vi "NI-DCPower Advanced Sequence Retrigger.vi"() -> ()   [LabVIEW 2023]
doc: "Demonstrates how to use the Advanced Sequence functions to change the output function in a sequence. This example initializes a session, configures the Source Delay, creates an Advanced Sequence, creates a step to set the configured Voltage Level in DC Voltage mode, creates a step to set the configured Current Level in DC Current mode, initiates generation, waits for a specified delay, and measures the voltage and current output. This example uses Advanced Sequence source mode."
uses:
  AdvancedSequenceSettings.ctl
  AdancedLCRSeqAppCluster.ctl
  MessageDef.ctl
  <instrlib>/niDCPower/nidcpower.llb/niDCPower Source Mode.ctl
  <instrlib>/niDCPower/nidcpower.llb/niDCPower Wait For Event - Event.ctl
  <instrlib>/niDCPower/nidcpower.llb/niDCPower Send Software Edge Trigger - Signal.ctl
  <instrlib>/niDCPower/nidcpower.llb/niDCPower Get Channel Name From String.vi
  <instrlib>/niDCPower/nidcpower.llb/niDCPower Configure Software Edge Start Trigger With Channels.vi
panel:
  in  "Combo Box":string(combo)="Mixed"
  in  "Trigger":bool
  in  "Stop":bool
  in  "Hardware timed Instrument Settings Inital Setup":T1[](array[typedef])=[{"Sequence Name"="LCRSweep_Low", "SequenceSettings"=[{"Instrument Mode"=1062, "LCR:AC Stimulus:Voltage Amplitude"=0.1, "LCR:AC Stimulus:Frequency"=1000.0, "Source:DC Voltage:Voltage Level"=0.0, "Source:DC Voltage:Current Limit"=0.001}, {"Instrument Mode"=1062, "LCR:AC Stimulus:Voltage Amplitude"=0.15, "LCR:AC Stimulus:Frequency"=2000.0, "Source:DC Voltage:Voltage Level"=0.0, "Source:DC Voltage:Current Limit"=0.001}, {"Instrument Mode"=1062, "LCR:AC Stimulus:Voltage Amplitude"=0.1, "LCR:AC Stimulus:Frequency"=2000.0, "Source:DC Voltage:Voltage Level"=0.0, "Source:DC Voltage:Current Limit"=1e-05}, {"Instrument Mode"=1062, "LCR:AC Stimulus:Voltage Amplitude"=0.1, "LCR:AC Stimulus:Frequency"=2000.0, "Source:DC Voltage:Voltage Level"=4.0, "Source:DC Voltage:Current Limit"=1e-05}, {"Instrument Mode"=1062, "LCR:AC Stimulus:Voltage Amplitude"=0.2, "LCR:AC Stimulus:Frequency"=2000.0, "Source:DC Voltage:Voltage Level"=3.0, "Source:DC Voltage:Current Limit"=1e-05}, {"Instrument Mode"=1062, "LCR:AC Stimulus:Voltage Amplitude"=1.0, "LCR:AC Stimulus:Frequency"=5000.0, "Source:DC Voltage:Voltage Level"=1.0, "Source:DC Voltage:Current Limit"=1e-05}]}, {"Sequence Name"="LCRSweep_High", "SequenceSettings"=[{"Instrument Mode"=1062, "LCR:AC Stimulus:Voltage Amplitude"=5.0, "LCR:AC Stimulus:Frequency"=1000.0, "Source:DC Voltage:Voltage Level"=0.0, "Source:DC Voltage:Current Limit"=0.001}, {"Instrument Mode"=1062, "LCR:AC Stimulus:Voltage Amplitude"=4.0, "LCR:AC Stimulus:Frequency"=2000.0, "Source:DC Voltage:Voltage Level"=0.0, "Source:DC Voltage:Current Limit"=0.001}, {"Instrument Mode"=1062, "LCR:AC Stimulus:Voltage Amplitude"=1.0, "LCR:AC Stimulus:Frequency"=2000.0, "Source:DC Voltage:Voltage Level"=0.0, "Source:DC Voltage:Current Limit"=1e-05}, {"Instrument Mode"=1062, "LCR:AC Stimulus:Voltage Amplitude"=1.5, "LCR:AC Stimulus:Frequency"=2000.0, "Source:DC Voltage:Voltage Level"=4.0, "Source:DC Voltage:Current Limit"=1e-05}, {"Instrument Mode"=1062, "LCR:AC Stimulus:Voltage Amplitude"=4.0, "LCR:AC Stimulus:Frequency"=2000.0, "Source:DC Voltage:Voltage Level"=3.0, "Source:DC Voltage:Current Limit"=1e-05}, {"Instrument Mode"=1062, "LCR:AC Stimulus:Voltage Amplitude"=3.0, "LCR:AC Stimulus:Frequency"=5000.0, "Source:DC Voltage:Voltage Level"=1.0, "Source:DC Voltage:Current Limit"=1e-05}]}, {"Sequence Name"="MixedModes", "SequenceSettings"=[{"Instrument Mode"=1062, "LCR:AC Stimulus:Voltage Amplitude"=1.0, "LCR:AC Stimulus:Frequency"=1000.0, "Source:DC Voltage:Voltage Level"=0.0, "Source:DC Voltage:Current Limit"=0.001}, {"Instrument Mode"=1061, "LCR:AC Stimulus:Voltage Amplitude"=0.15, "LCR:AC Stimulus:Frequency"=2000.0, "Source:DC Voltage:Voltage Level"=3.0, "Source:DC Voltage:Current Limit"=0.001}, {"Instrument Mode"=1062, "LCR:AC Stimulus:Voltage Amplitude"=1.0, "LCR:AC Stimulus:Frequency"=2000.0, "Source:DC Voltage:Voltage Level"=0.0, "Source:DC Voltage:Current Limit"=1e-05}, {"Instrument Mode"=1061, "LCR:AC Stimulus:Voltage Amplitude"=0.1, "LCR:AC Stimulus:Frequency"=2000.0, "Source:DC Voltage:Voltage Level"=2.0, "Source:DC Voltage:Current Limit"=1e-05}, {"Instrument Mode"=1062, "LCR:AC Stimulus:Voltage Amplitude"=0.2, "LCR:AC Stimulus:Frequency"=2000.0, "Source:DC Voltage:Voltage Level"=3.0, "Source:DC Voltage:Current Limit"=1e-05}, {"Instrument Mode"=1062, "LCR:AC Stimulus:Voltage Amplitude"=1.0, "LCR:AC Stimulus:Frequency"=5000.0, "Source:DC Voltage:Voltage Level"=1.0, "Source:DC Voltage:Current Limit"=1e-05}]}, {"Sequence Name"="SMU_Low", "SequenceSettings"=[{"Instrument Mode"=1062, "LCR:AC Stimulus:Voltage Amplitude"=0.1, "LCR:AC Stimulus:Frequency"=1000.0, "Source:DC Voltage:Voltage Level"=0.0, "Source:DC Voltage:Current Limit"=0.001}, {"Instrument Mode"=1062, "LCR:AC Stimulus:Voltage Amplitude"=0.15, "LCR:AC Stimulus:Frequency"=2000.0, "Source:DC Voltage:Voltage Level"=1.0, "Source:DC Voltage:Current Limit"=0.001}, {"Instrument Mode"=1062, "LCR:AC Stimulus:Voltage Amplitude"=0.1, "LCR:AC Stimulus:Frequency"=2000.0, "Source:DC Voltage:Voltage Level"=0.0, "Source:DC Voltage:Current Limit"=1e-05}, {"Instrument Mode"=1062, "LCR:AC Stimulus:Voltage Amplitude"=0.1, "LCR:AC Stimulus:Frequency"=2000.0, "Source:DC Voltage:Voltage Level"=2.0, "Source:DC Voltage:Current Limit"=1e-05}, {"Instrument Mode"=1061, "LCR:AC Stimulus:Voltage Amplitude"=0.2, "LCR:AC Stimulus:Frequency"=2000.0, "Source:DC Voltage:Voltage Level"=1.0, "Source:DC Voltage:Current Limit"=1e-05}, {"Instrument Mode"=1062, "LCR:AC Stimulus:Voltage Amplitude"=1.0, "LCR:AC Stimulus:Frequency"=5000.0, "Source:DC Voltage:Voltage Level"=1.0, "Source:DC Voltage:Current Limit"=1e-05}]}, {"Sequence Name"="SMU_High", "SequenceSettings"=[{"Instrument Mode"=1062, "LCR:AC Stimulus:Voltage Amplitude"=0.1, "LCR:AC Stimulus:Frequency"=1000.0, "Source:DC Voltage:Voltage Level"=3.0, "Source:DC Voltage:Current Limit"=0.001}, {"Instrument Mode"=1061, "LCR:AC Stimulus:Voltage Amplitude"=0.15, "LCR:AC Stimulus:Frequency"=2000.0, "Source:DC Voltage:Voltage Level"=2.0, "Source:DC Voltage:Current Limit"=0.001}, {"Instrument Mode"=1062, "LCR:AC Stimulus:Voltage Amplitude"=0.1, "LCR:AC Stimulus:Frequency"=2000.0, "Source:DC Voltage:Voltage Level"=6.0, "Source:DC Voltage:Current Limit"=1e-05}, {"Instrument Mode"=1062, "LCR:AC Stimulus:Voltage Amplitude"=0.1, "LCR:AC Stimulus:Frequency"=2000.0, "Source:DC Voltage:Voltage Level"=10.0, "Source:DC Voltage:Current Limit"=1e-05}, {"Instrument Mode"=1062, "LCR:AC Stimulus:Voltage Amplitude"=0.2, "LCR:AC Stimulus:Frequency"=2000.0, "Source:DC Voltage:Voltage Level"=7.0, "Source:DC Voltage:Current Limit"=1e-05}, {"Instrument Mode"=1062, "LCR:AC Stimulus:Voltage Amplitude"=1.0, "LCR:AC Stimulus:Frequency"=5000.0, "Source:DC Voltage:Voltage Level"=8.0, "Source:DC Voltage:Current Limit"=1e-05}]}, {"Sequence Name"="MixedMode_2", "SequenceSettings"=[{"Instrument Mode"=1062, "LCR:AC Stimulus:Voltage Amplitude"=0.1, "LCR:AC Stimulus:Frequency"=1000.0, "Source:DC Voltage:Voltage Level"=0.0, "Source:DC Voltage:Current Limit"=0.001}, {"Instrument Mode"=1062, "LCR:AC Stimulus:Voltage Amplitude"=0.15, "LCR:AC Stimulus:Frequency"=2000.0, "Source:DC Voltage:Voltage Level"=0.0, "Source:DC Voltage:Current Limit"=0.001}, {"Instrument Mode"=1061, "LCR:AC Stimulus:Voltage Amplitude"=0.1, "LCR:AC Stimulus:Frequency"=2000.0, "Source:DC Voltage:Voltage Level"=0.0, "Source:DC Voltage:Current Limit"=1e-05}, {"Instrument Mode"=1062, "LCR:AC Stimulus:Voltage Amplitude"=0.1, "LCR:AC Stimulus:Frequency"=2000.0, "Source:DC Voltage:Voltage Level"=4.0, "Source:DC Voltage:Current Limit"=1e-05}, {"Instrument Mode"=1061, "LCR:AC Stimulus:Voltage Amplitude"=0.2, "LCR:AC Stimulus:Frequency"=2000.0, "Source:DC Voltage:Voltage Level"=3.0, "Source:DC Voltage:Current Limit"=1e-05}, {"Instrument Mode"=1062, "LCR:AC Stimulus:Voltage Amplitude"=1.0, "LCR:AC Stimulus:Frequency"=5000.0, "Source:DC Voltage:Voltage Level"=1.0, "Source:DC Voltage:Current Limit"=1e-05}]}] {"SequenceSettings"."Instrument Mode" items=["SMU PS"=1061, "LCR"=1062, "E-Load"=1154]}
  out "error out":errorcluster
  out "Data":T2(graph)
  in  "Resource Name":refnum<k15>="SMU_4139_C02_S02"
  # "This Demo shows the reuse of Advanced Hardware timed sequences. In the Array on the left side the Sequences are defined and loaded\nWhile the Application is running you can then trigger these Sequences by Selecting the Sequence in the Combobox and press the Trigger Button."
  # "Init Application"
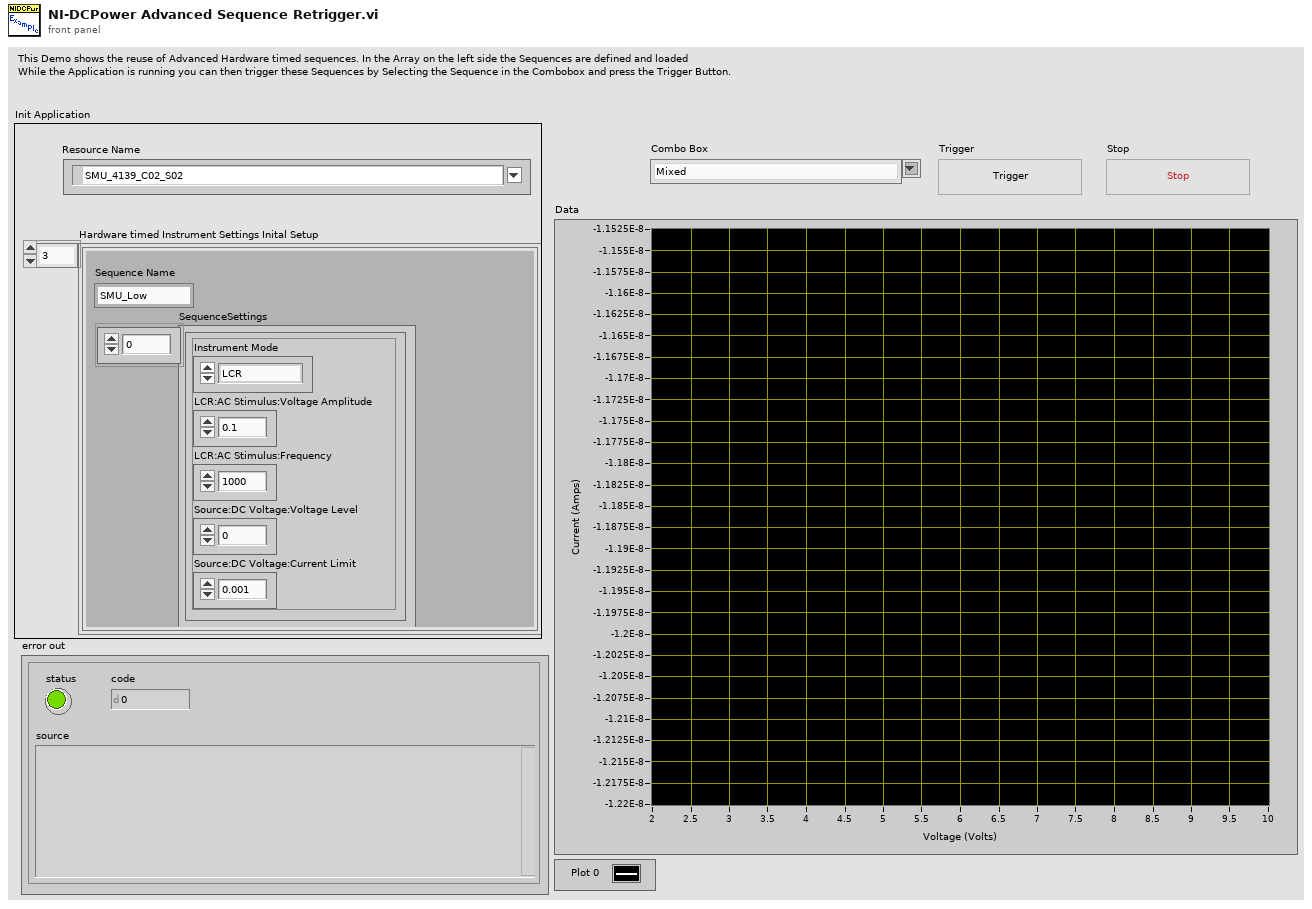
[diagram p1: front panel]
types:
  T1 = typedef "AdvancedSequenceSettings.ctl" = cluster{"Sequence Name":string, "SequenceSettings":cluster{"Instrument Mode":i32, "LCR:AC Stimulus:Voltage Amplitude":dbl, "LCR:AC Stimulus:Frequency":dbl, "Source:DC Voltage:Voltage Level":dbl, "Source:DC Voltage:Current Limit":dbl}[]}
  T2 = cluster{"voltage measurements":dbl[], "current measurements":dbl[]}
  T3 = typedef "AdancedLCRSeqAppCluster.ctl" = cluster{"queue out":refnum<queue>, "sequence name":string[], "Channelname":string, "instrument handle out":refnum<k15>}
  T4 = typedef "MessageDef.ctl" = cluster{"Message":string, "Data":variant}
  T5 = typedef "niDCPower Source Mode.ctl" = i32
  T6 = typedef "niDCPower Send Software Edge Trigger - Signal.ctl" = i32
  T7 = typedef "niDCPower Wait For Event - Event.ctl" = i32
  T8 = cluster{"Instrument Mode":i32, "LCR:AC Stimulus:Voltage Amplitude":dbl, "LCR:AC Stimulus:Frequency":dbl, "Source:DC Voltage:Voltage Level":dbl, "Source:DC Voltage:Current Limit":dbl}[]
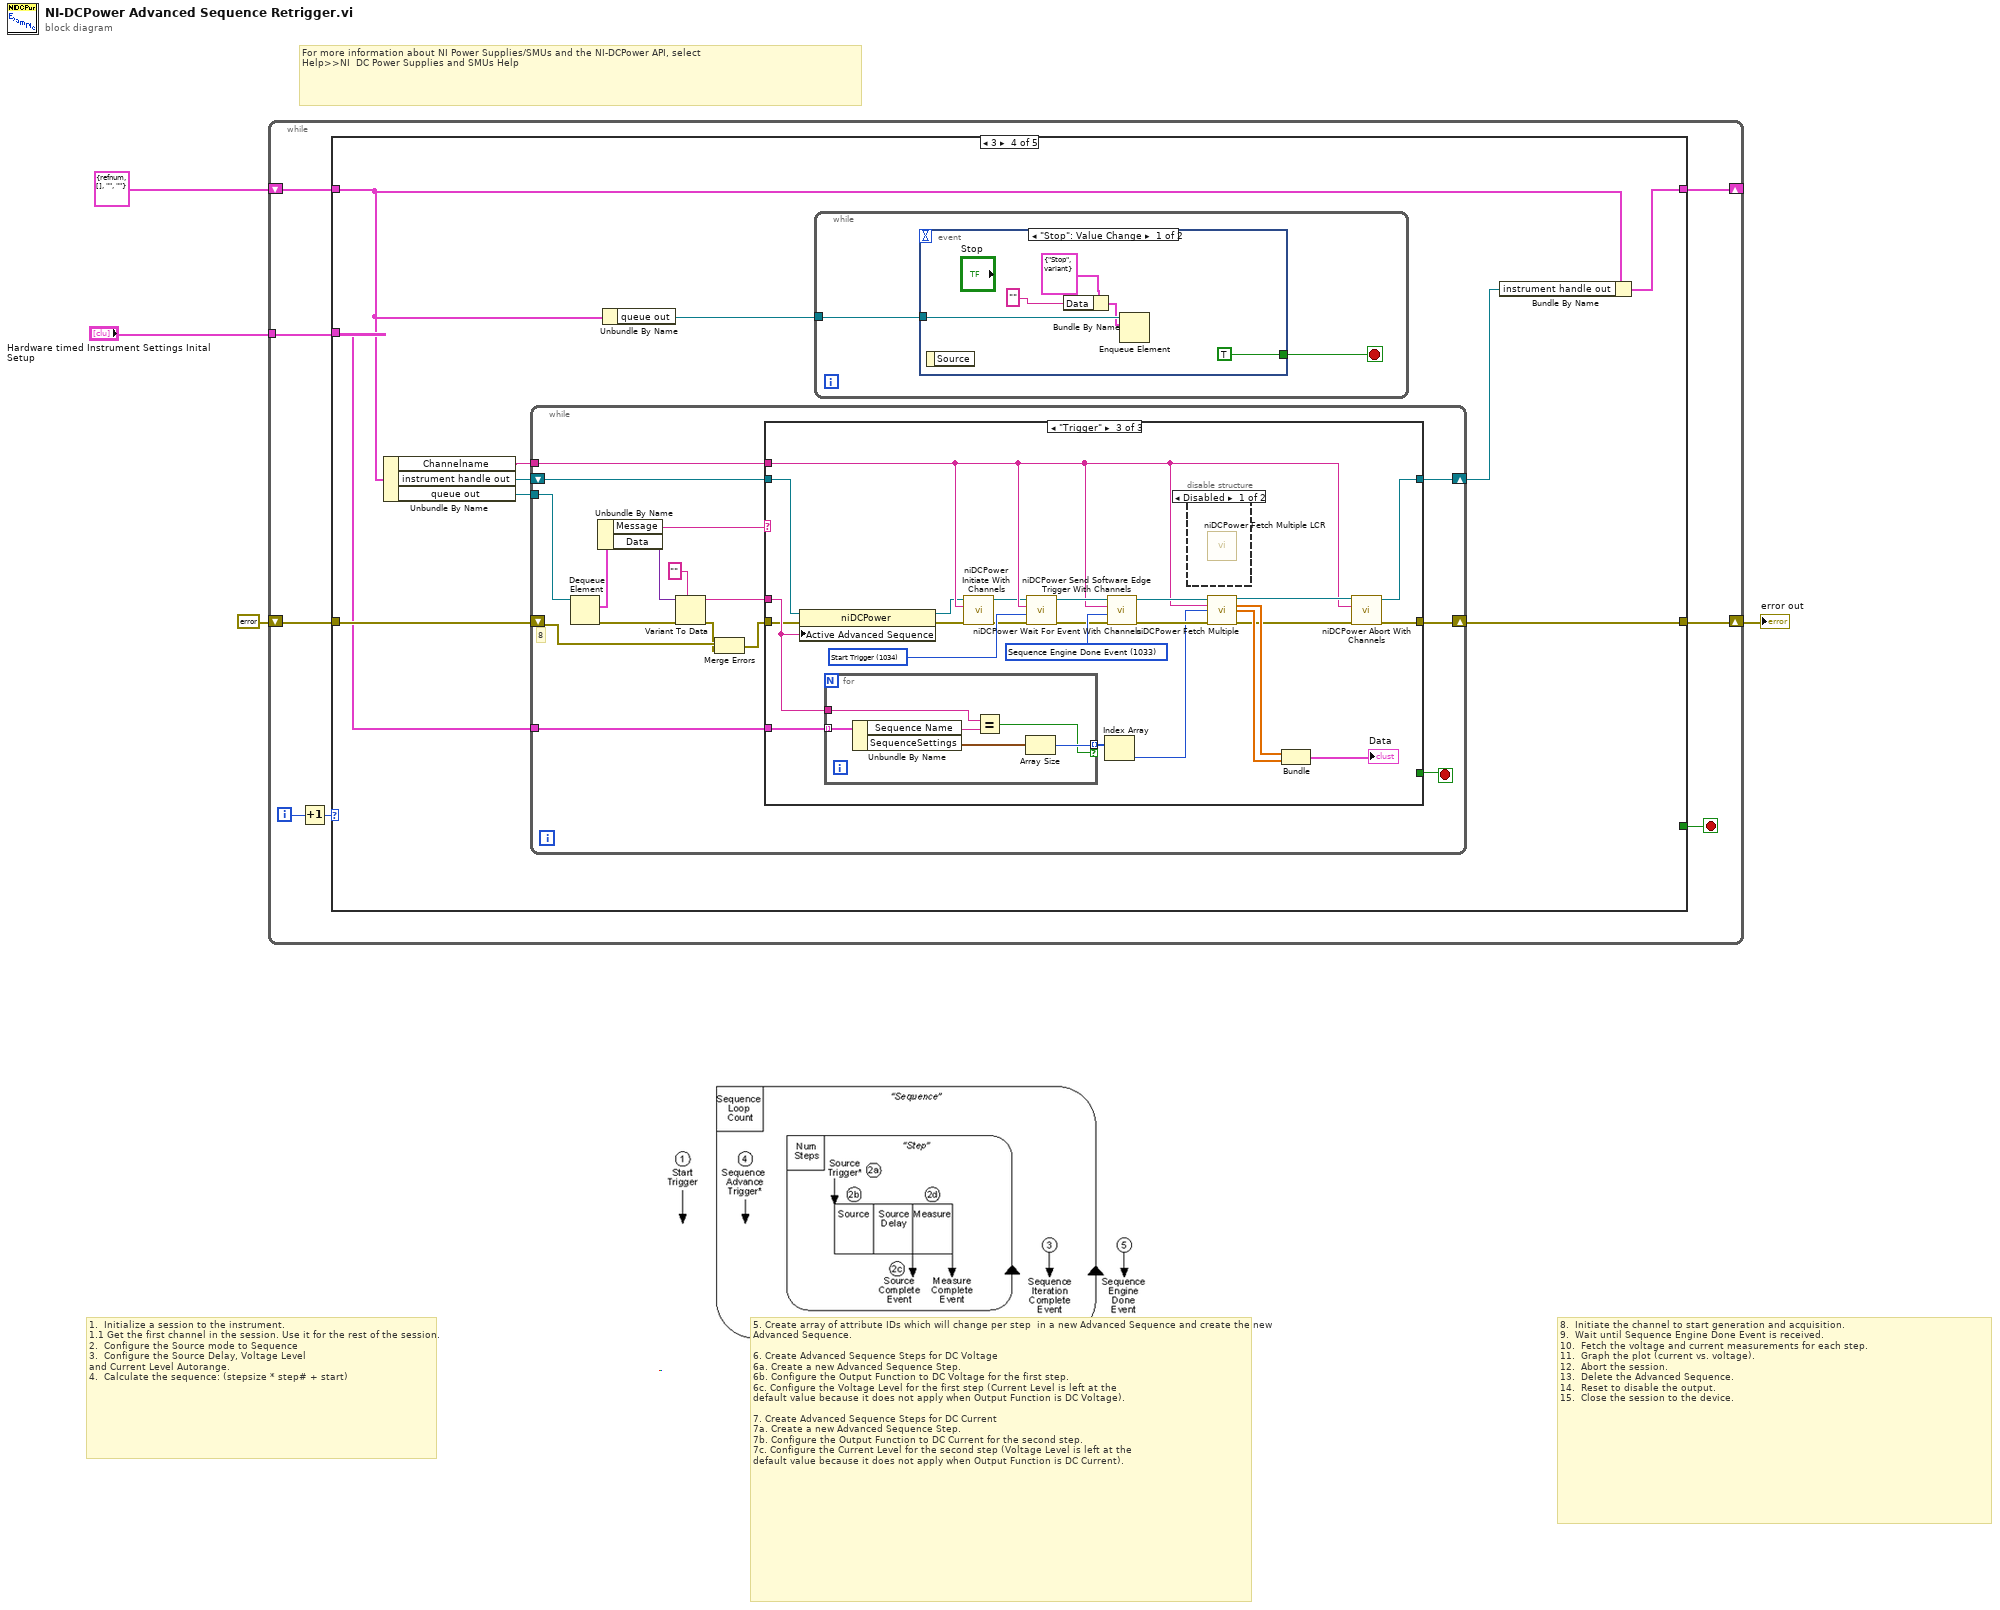
[diagram p0: block diagram]
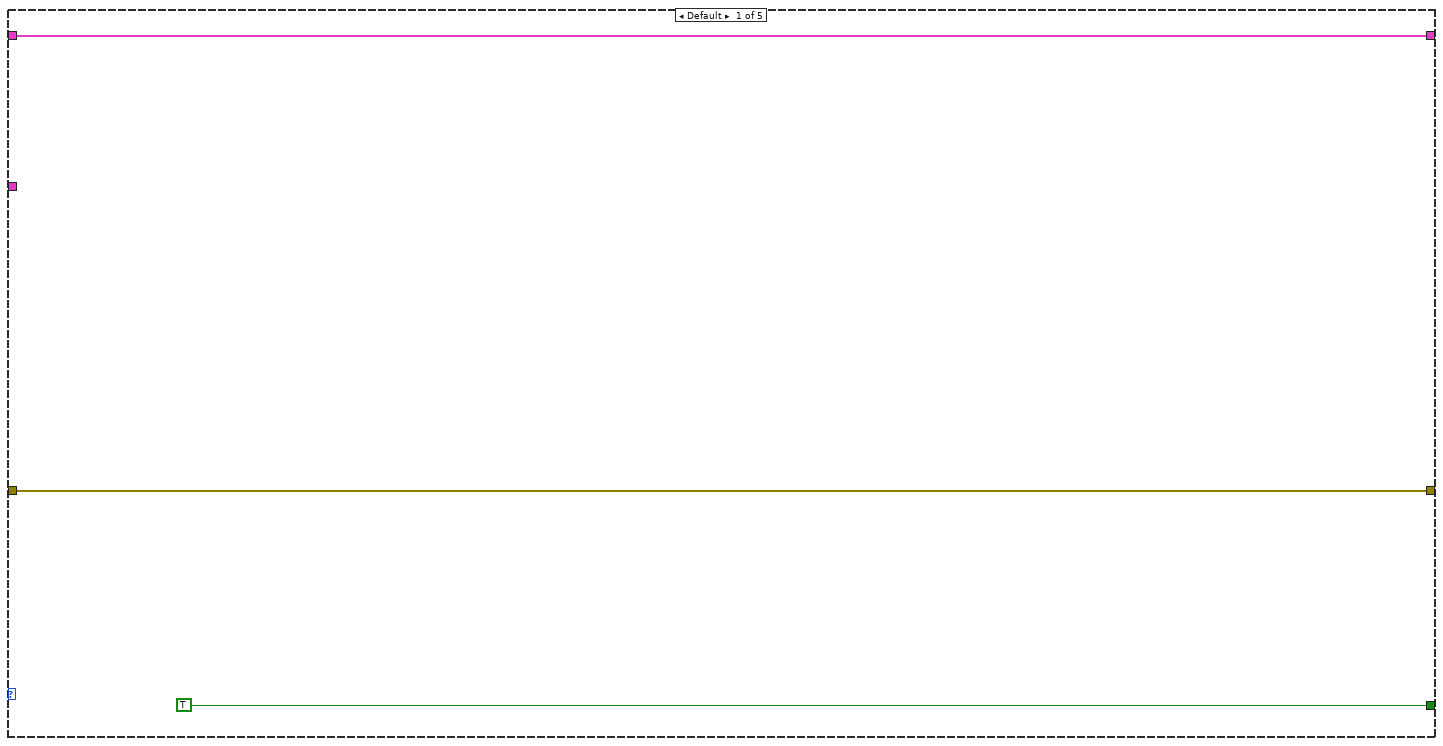
[diagram p2: hidden frame]
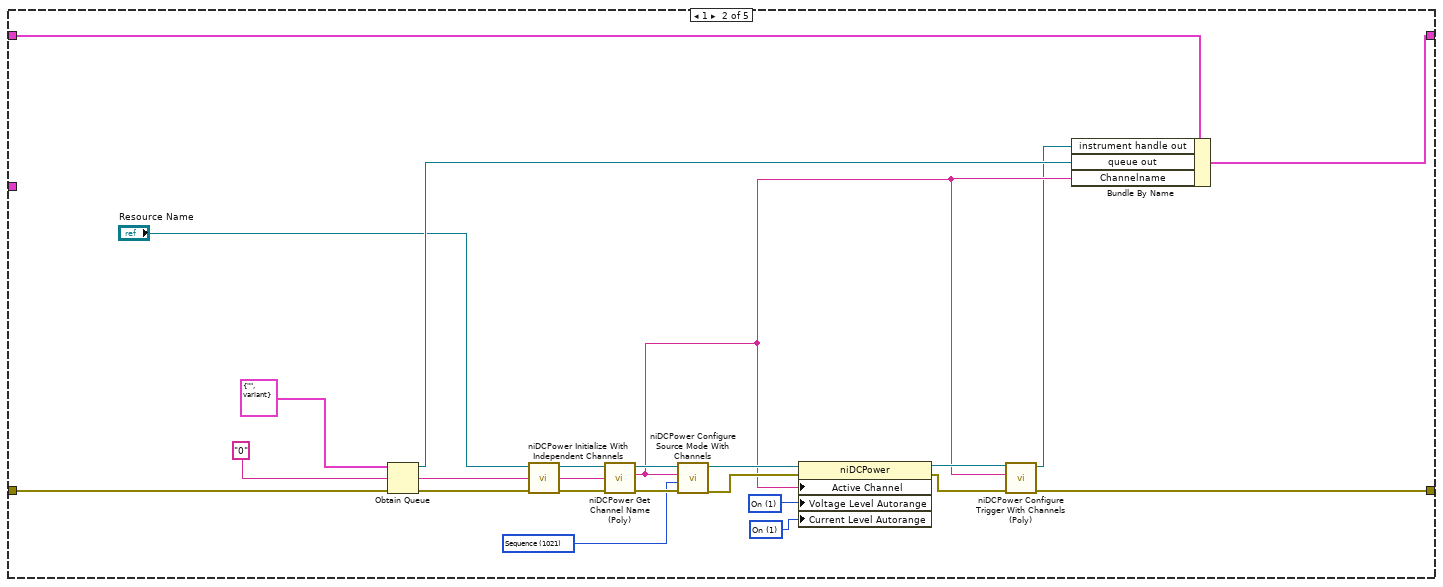
[diagram p3: hidden frame]
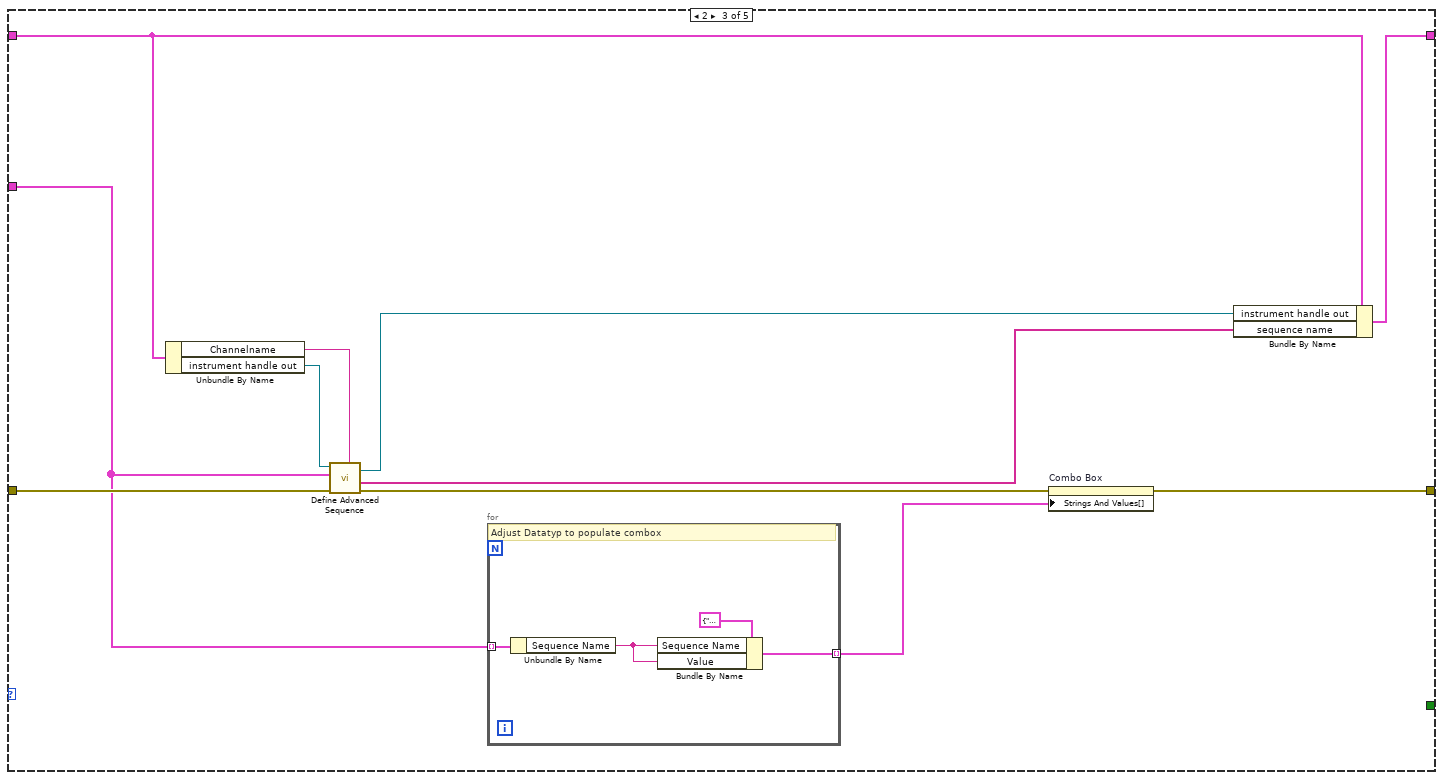
[diagram p4: hidden frame]
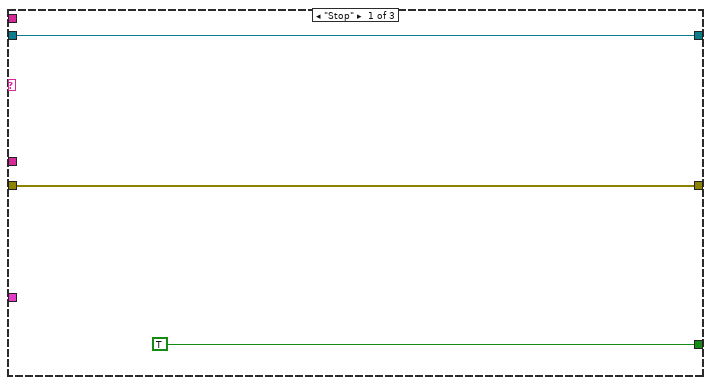
[diagram p5: hidden frame]
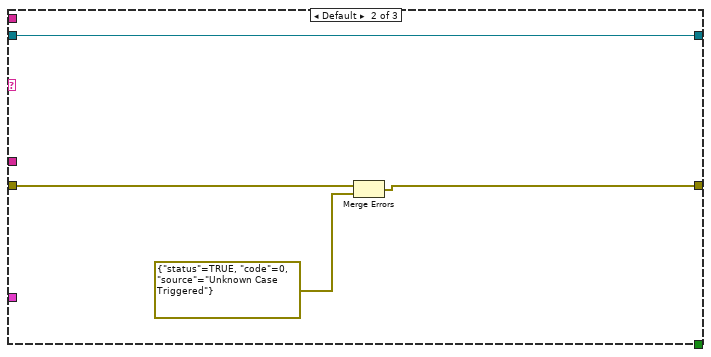
[diagram p6: hidden frame]
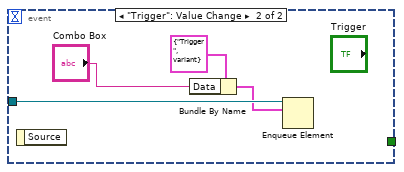
[diagram p8: hidden frame]
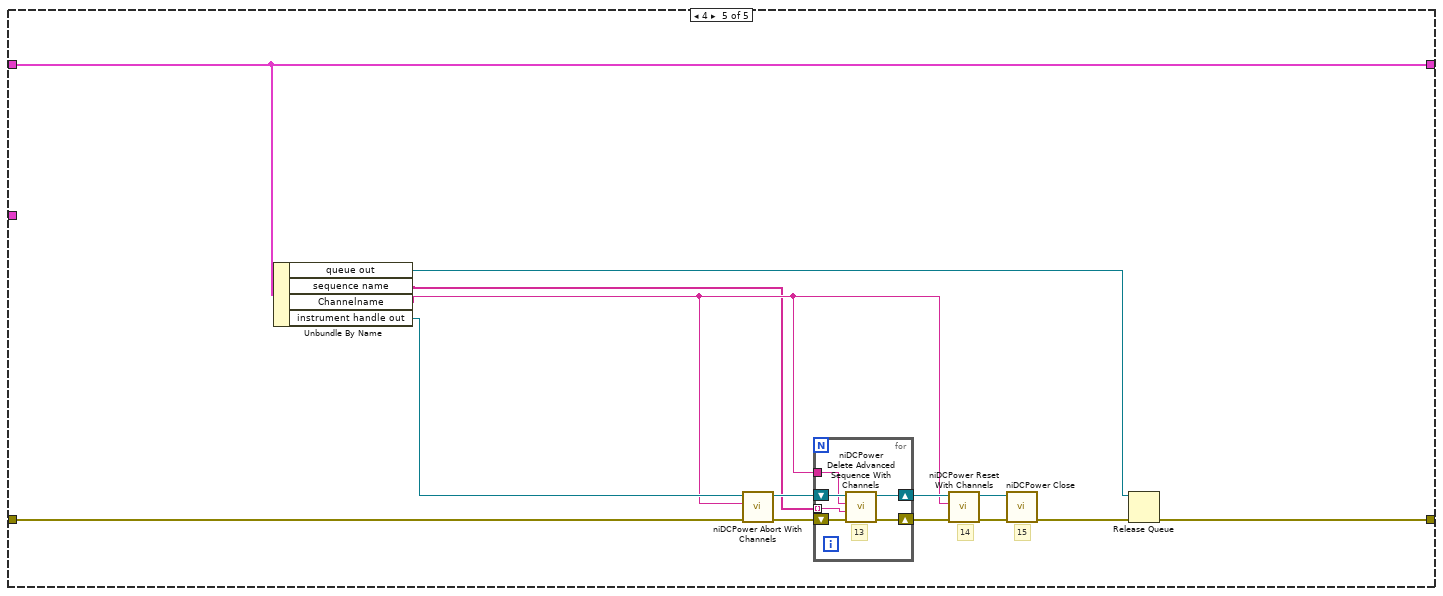
[diagram p9: hidden frame]
diagram:
  # "8.  Initiate the channel to start generation and acquisition.\n9.  Wait until Sequence Engine Done Event is received.\n10.  Fetch the voltage and current measurements for each step.\n11.  Graph the plot (current vs. voltage).\n12.  Abort the session.\n13.  Delete the Advanced Sequence.\n14.  Reset to disable the output.\n15.  Close the session to the device."
  # "For more information about NI Power Supplies/SMUs and the NI-DCPower API, select\nHelp>>NI  DC Power Supplies and SMUs Help"
  # "1.  Initialize a session to the instrument.\n1.1 Get the first channel in the session. Use it for the rest of the session.\n2.  Configure the Source mode to Sequence\n3.  Configure the Source Delay, Voltage Level\nand Current Level Autorange.\n4.  Calculate the sequence: (stepsize * step# + start)"
  # "5. Create array of attribute IDs which will change per step  in a new Advanced Sequence and create the new Advanced Sequence.\n\n6. Create Advanced Sequence Steps for DC Voltage\n6a. Create a new Advanced Sequence Step.\n6b. Configure the Output Function to DC Voltage for the first step.\n6c. Configure the Voltage Level for the first step (Current Level is left at the\ndefault value because it does not apply when Output Function is DC Voltage).\n\n7. Create Advanced Sequence Steps for DC Current\n7a. Create a new Advanced Sequence Step.\n7b. Configure the Output Function to DC Current for the second step.\n7c. Configure the Current Level for the second step (Voltage Level is left at the\ndefault value because it does not apply when Output Function is DC Current)."
  n1 = while {
    shift-right: [w8] -> w4
    shift-left: errorcluster {"status"=FALSE, "code"=0, "source"=""} ("error out") -> [w12]
    tunnel: "Hardware timed Instrument Settings Inital Setup" -> [w7]
    shift-right: [w5] -> _
    shift-left: T3 {"queue out"=refnum, "sequence name"=[], "Channelname"="", "instrument handle out"=""} -> [w6]
    i -> [w11]
    stop <- w9 stop-if-true
    n2 = Increment(x=w11) -> (x+1=w10:i32)
    n3 = case shown="3" w10 {
      tunnel: [w14 w25 w41 w62 w132] -> w8
      tunnel: w12 -> [w14 w24 w48 w61 w134]
      tunnel: [TRUE _ _ _ _] -> w9
      tunnel: w7 -> [_ _ w39 w53 _]
      tunnel: w6 -> [w13 w22 w46 w55 w131]
      tunnel: [w13 w19 w45 w56 w131] -> w5
      frame Default {
      }
      frame 1 {
        w32 = 1 items=["Off", "On"] ("Source:DC Current:Current Level Autorange")
        w33 = 1 items=["Off", "On"] ("Source:DC Voltage:Voltage Level Autorange")
        w30 = T5 1021 items=["Single Point"=1020, "Sequence"=1021] ("source mode")
        n4 = Obtain Queue(element data type=T4 {"Message"="", "Data"=variant} ("Message"), error in (no error)=w24) -> (queue out=w21:refnum<queue>, error out=w23:errorcluster)  [unwired: 3 in, 1 out]
        n5 = call <instrlib>:"niDCPower Initialize With Independent Channels.vi"("error in (no error)"=w23, "resource name"="Resource Name") -> ("error out"=w35:errorcluster, "instrument handle out"=w29:refnum<k15>)  [unwired: 8 in]
        n6 = call-poly <instrlib>:"niDCPower Get Channel Name (Poly).vi"("error in (no error)"=w35, "index"="0", "instrument handle"=w29) -> ("error out"=w36:errorcluster, "name"=w20:string, "instrument handle out"=w28:refnum<k15>)  [unwired: 6 in]
        n7 = call <instrlib>:"niDCPower Configure Source Mode With Channels.vi"("error in (no error)"=w36, "source mode"=w30, "channel name"=w20, "instrument handle"=w28) -> ("error out"=w34:errorcluster, "instrument handle out"=w27:refnum<k15>)  [unwired: 6 in]
        n8 = property class="niDCPower"(reference=w27, error in=w34, "Active Channel"=w20, "Voltage Level Autorange"=w33, "Current Level Autorange"=w32) -> (reference out=w26:refnum<k15>, error out=w37:errorcluster)
        n9 = call-poly <instrlib>:"niDCPower Configure Trigger With Channels (Poly).vi"("error in (no error)"=w37, "channel name"=w20, "instrument handle"=w26) -> ("error out"=w25:errorcluster, "instrument handle out"=w18:refnum<k15>)  [unwired: 7 in]
        n10 = Bundle By Name(cluster=w22, "instrument handle out"=w18, "queue out"=w21, "Channelname"=w20) -> (w19:T3)
      }
      frame 2 {
        n11 = Unbundle By Name(w46) -> ("Channelname"=w44:string, "instrument handle out"=w47:refnum<k15>)
        n12 = call "Define Advanced Sequence.vi"("ChannelName"=w44, "error in (no error)"=w48, "Hardware timed Instrument Settings"=w39, "IVI Refnum in"=w47) -> ("error out"=w42:errorcluster, "sequence name"=w40:string[], "IVI Refnum out"=w43:refnum<k15>)  [unwired: 5 in]
        n13 = for {
          tunnel: w39 -> [w52] mode=indexing
          tunnel: [w50] -> w38 mode=indexing
          # "Adjust Datatyp to populate combox"
          n14 = Unbundle By Name(w52) -> ("Sequence Name"=w49:string)
          n15 = Bundle By Name(cluster=cluster{"Sequence Name":string, "Value":string} {"Sequence Name"="", "Value"=""}, "Sequence Name"=w49, "Value"=w49) -> (w50:cluster{"Sequence Name":string, "Value":string})
        }
        n16 = property on="Combo Box" class="CmbBox"(error in=w42, "Strings And Values[]"=w38) -> (error out=w41:errorcluster)  [unwired: 1 in, 1 out]
        n17 = Bundle By Name(cluster=w46, "instrument handle out"=w43, "sequence name"=w40) -> (w45:T3)
      }
      frame 3 {
        n18 = Unbundle By Name(w55) -> ("Channelname"=w58:string, "instrument handle out"=w59:refnum<k15>, "queue out"=w60:refnum<queue>)
        n19 = while {
          shift-right: [w78] -> w62
          shift-left: w61 -> [w70]
          tunnel: w60 -> [w76]
          tunnel: w58 -> [w74]
          shift-right: [w73] -> w57
          shift-left: w59 -> [w75]
          tunnel: w53 -> [w68]
          stop <- w71 stop-if-true
          # "8"
          n20 = Dequeue Element(queue=w76) -> (element=w77:T4, error out=w67:errorcluster)  [unwired: 2 in, 2 out]
          n21 = Unbundle By Name(w77) -> ("Message"=w72:string, "Data"=w64:variant)
          n22 = Variant To Data(error in=w67, type="" ("Message"), Variant=w64) -> (data=w63:string, error out=w66:errorcluster)
          n23 = Merge Errors(w70, w66) -> (w69:errorcluster)
          n24 = case shown="\"Trigger\"" w72 {
            tunnel: w69 -> [w80 w84 w87]
            tunnel: [w80 w83 w91] -> w78
            tunnel: [w79 w85 w92] -> w73
            tunnel: w75 -> [w79 w85 w90]
            tunnel: w74 -> [_ _ w95]
            tunnel: [TRUE _ _] -> w71
            tunnel: w68 -> [_ _ w98]
            tunnel: w63 -> [_ _ w88]
            frame "Stop" {
            }
            frame Default {
              n25 = Merge Errors(w84, errorcluster {"status"=TRUE, "code"=0, "source"="Unknown Case Triggered"} ("error in")) -> (w83:errorcluster)
            }
            frame "Trigger" {
              w102 = T6 1034 items=["Start Trigger"=1034, "Source Trigger"=1035, "Measure Trigger"=1036, "Sequence Advance Trigger"=1037, "Pulse Trigger"=1053, "Shutdown Trigger"=1118] ("signal")
              w107 = T7 1033 items=["Source Complete Event"=1030, "Measure Complete Event"=1031, "Sequence Iteration Complete Event"=1032, "Sequence Engine Done Event"=1033] ("event")
              n26 = property class="niDCPower"(reference=w90, error in=w87, "Active Advanced Sequence"=w88) -> (reference out=w89:refnum<k15>, error out=w86:errorcluster)
              n27 = for {
                tunnel: w98 -> [w115] mode=indexing
                tunnel: w88 -> [w113]
                tunnel: [w111] -> w97 mode=indexing if=w110
                n28 = Unbundle By Name(w115) -> ("Sequence Name"=w114:string, "SequenceSettings"=w112:T8)
                n29 = Equal?(x=w113, y=w114) -> (x = y?=w110:bool)
                n30 = Array Size(array=w112) -> (size(s)=w111:i32)
              }
              n31 = call <instrlib>:"niDCPower Initiate With Channels.vi"("error in (no error)"=w86, "channel name"=w95, "instrument handle"=w89) -> ("error out"=w94:errorcluster, "instrument handle out"=w93:refnum<k15>)  [unwired: 7 in]
              n32 = call <instrlib>:"niDCPower Send Software Edge Trigger With Channels.vi"("error in (no error)"=w94, "signal"=w102, "channel name"=w95, "instrument handle"=w93) -> ("error out"=w104:errorcluster, "instrument handle out"=w103:refnum<k15>)  [unwired: 6 in]
              n33 = Index Array(array=w97) -> (element=w96:i32)  [unwired: 1 in]
              n34 = call <instrlib>:"niDCPower Wait For Event With Channels.vi"("error in (no error)"=w104, "event"=w107, "channel name"=w95, "instrument handle"=w103) -> ("error out"=w108:errorcluster, "instrument handle out"=w109:refnum<k15>)  [unwired: 6 in]
              n35 = disable-structure shown="Disabled" {
                frame Disabled {
                  n36 = call <instrlib>:"niDCPower Fetch Multiple LCR.vi"() -> ()  [unwired: 12 in, 4 out]
                }
                frame Enabled {
                }
              }
              n37 = call <instrlib>:"niDCPower Fetch Multiple.vi"("instrument handle"=w109, "channel name"=w95, "count (1)"=w96, "error in (no error)"=w108) -> ("instrument handle out"=w100:refnum<k15>, "voltage measurements"=w106:dbl[], "current measurements"=w105:dbl[], "error out"=w101:errorcluster)  [unwired: 6 in, 2 out]
              n38 = Bundle("voltage measurements"=w106, "current measurements"=w105) -> (→"Data":T2)  [unwired: 1 out]
              n39 = call <instrlib>:"niDCPower Abort With Channels.vi"("error in (no error)"=w101, "channel name"=w95, "instrument handle"=w100) -> ("error out"=w91:errorcluster, "instrument handle out"=w92:refnum<k15>)  [unwired: 7 in]
            }
          }
        }
        n40 = Unbundle By Name(w55) -> ("queue out"=w54:refnum<queue>)
        n41 = while {
          tunnel: w54 -> [w116]
          stop <- w117 stop-if-true
          n42 = event shown="[0] \"Stop\": Value Change" {
            selector: _ -> [_ _]
            dyn-events: _ -> [_ _]
            timeout: _ -> [_ _]
            tunnel: [TRUE _] -> w117
            tunnel: w116 -> [w121 w126]
            event "Stop": Value Change {
              n43 = event-data() -> ()  [unwired: 1 in, 1 out]
              n44 = Bundle By Name(cluster=T4 {"Message"="Stop", "Data"=variant} ("element"), "Data"="" ("Message")) -> (w119:T4)
              n45 = Enqueue Element(queue=w121, element=w119) -> ()  [unwired: 2 in, 3 out]
            }
            event "Trigger": Value Change {
              n46 = event-data() -> ()  [unwired: 1 in, 1 out]
              n47 = Bundle By Name(cluster=T4 {"Message"="Trigger", "Data"=variant} ("element"), "Data"="Combo Box") -> (w124:T4)
              n48 = Enqueue Element(queue=w126, element=w124) -> ()  [unwired: 2 in, 3 out]
            }
          }
        }
        n49 = Bundle By Name(cluster=w55, "instrument handle out"=w57) -> (w56:T3)
      }
      frame 4 {
        # "15"
        # "14"
        n50 = Unbundle By Name(w131) -> ("queue out"=w130:refnum<queue>, "sequence name"=w127:string[], "Channelname"=w128:string, "instrument handle out"=w129:refnum<k15>)
        n51 = call <instrlib>:"niDCPower Abort With Channels.vi"("error in (no error)"=w134, "channel name"=w128, "instrument handle"=w129) -> ("error out"=w139:errorcluster, "instrument handle out"=w140:refnum<k15>)  [unwired: 7 in]
        n52 = for {
          shift-right: [w146] -> w137
          shift-left: w139 -> [w144]
          shift-right: [w145] -> w138
          shift-left: w140 -> [w143]
          tunnel: w128 -> [w142]
          tunnel: w127 -> [w141] mode=indexing
          # "13"
          n53 = call <instrlib>:"niDCPower Delete Advanced Sequence With Channels.vi"("error in (no error)"=w144, "sequence name"=w141, "channel name"=w142, "instrument handle"=w143) -> ("error out"=w146:errorcluster, "instrument handle out"=w145:refnum<k15>)  [unwired: 6 in]
        }
        n54 = call <instrlib>:"niDCPower Reset With Channels.vi"("error in (no error)"=w137, "channel name"=w128, "instrument handle"=w138) -> ("error out"=w136:errorcluster, "instrument handle out"=w135:refnum<k15>)  [unwired: 7 in]
        n55 = call <instrlib>:"niDCPower Close.vi"("error in (no error)"=w136, "instrument handle"=w135) -> ("error out"=w133:errorcluster)  [unwired: 9 out]
        n56 = Release Queue(queue=w130, error in (no error)=w133) -> (error out=w132:errorcluster)  [unwired: 1 in, 2 out]
      }
    }
  }
  "error out" <- w4
